vi "goto2.vi"() -> ()   [LabVIEW 2016]
uses:
  <vilib>/addons/control/pid/pid.llb/PID (DBL).vi
  <vilib>/addons/control/pid/NI_PID_pid.lvlib
panel:
  in  "max pwm\ndist condition":dbl=500.0 format="%#_13g"
  in  "max  pwm\nmultiplier":dbl=1.0 format="%#_13g"
  in  "stop dist\ncondition":dbl=100.0 format="%#_13g"
  in  "PID gains":T1={"proportional gain (Kc)"=1.0, "integral time (Ti, min)"=0.01, "derivative time (Td, min)"=0.0} {"derivative time (Td, min)" format="%.3f"; "integral time (Ti, min)" format="%.3f"; "proportional gain (Kc)" format="%.3f"}
  in  "gain":dbl=0.01 format="%#_13g"
  out "speed out":dbl[](array[numeric])
  in  "Pose":dbl[](array[numeric])
  in  "Target":dbl[](array[numeric])
  # "X"
  # "Y"
  # "W"
  # "X"
  # "vx"
  # "Y"
  # "vy"
  # "W"
  # "vw"
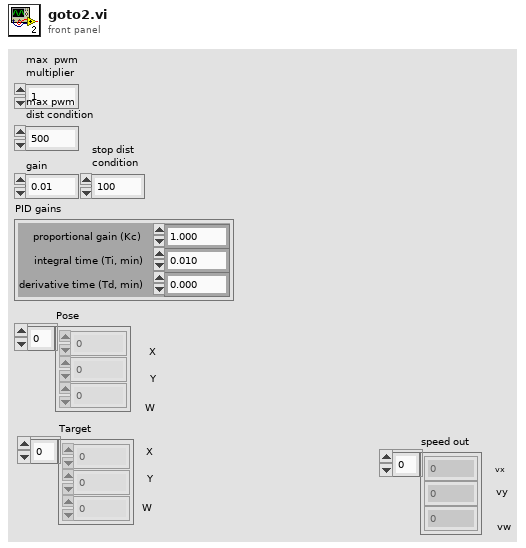
[diagram p1: front panel]
types:
  T1 = cluster{"proportional gain (Kc)":dbl, "integral time (Ti, min)":dbl, "derivative time (Td, min)":dbl}
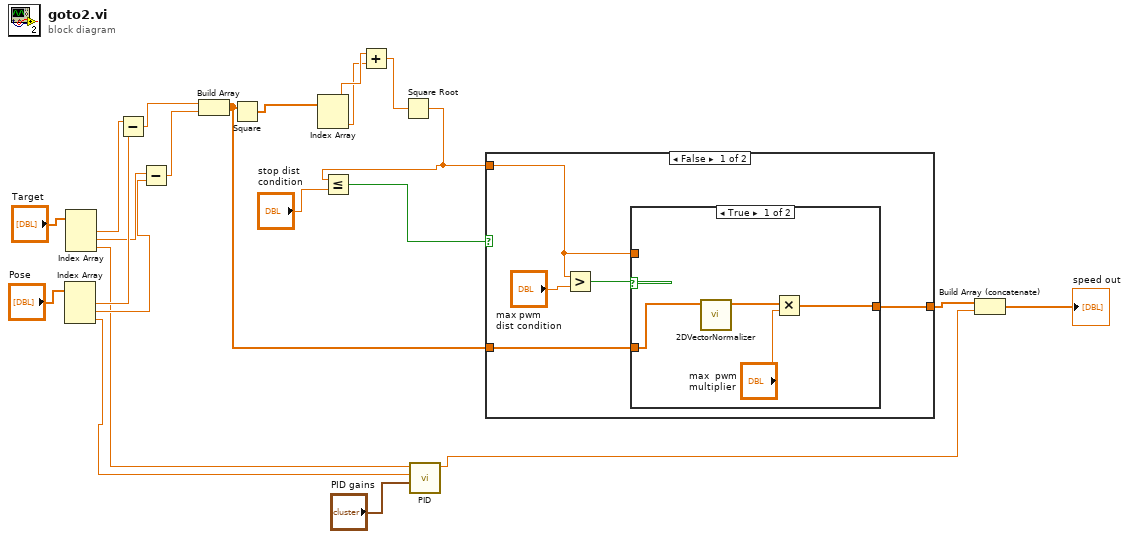
[diagram p0: block diagram]
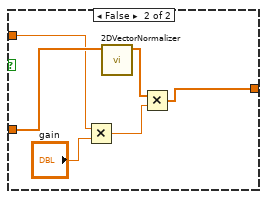
[diagram p2: hidden frame]
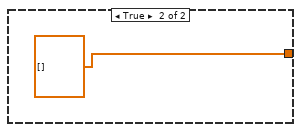
[diagram p3: hidden frame]
diagram:
  n1 = Index Array(array="Pose") -> (element #1=w19:dbl, element #2=w17:dbl, element #3=w5:dbl)  [unwired: 3 in]
  n2 = Index Array(array="Target") -> (element #1=w20:dbl, element #2=w18:dbl, element #3=w6:dbl)  [unwired: 3 in]
  n3 = Subtract(x=w20, y=w19) -> (x-y=w13:dbl)
  n4 = Subtract(x=w18, y=w17) -> (x-y=w14:dbl)
  n5 = Build Array(w13, w14) -> (w10:dbl[])
  n6 = Square(x=w10) -> (x^2=w9:dbl[])
  n7 = Index Array(array=w9) -> (element #1=w12:dbl, element #2=w11:dbl)  [unwired: 2 in]
  n8 = Add(x=w12, y=w11) -> (x+y=w8:dbl)
  n9 = Square Root(x=w8) -> (sqrt(x)=w7:dbl)
  n10 = Less Or Equal?(x=w7, y="stop dist\ncondition") -> (x <= y?=w15:bool)
  n11 = call-poly <vilib>:"PID.vi"("PID gains"="PID gains", "process variable"=w5, "setpoint"=w6) -> ("output"=w2:dbl)  [unwired: 7 in, 1 out]
  n12 = case shown="False" w15 {
    tunnel: w7 -> [w24 _]
    tunnel: [w23 dbl[] [] ("appended array")] -> w3
    tunnel: w10 -> [w25 _]
    frame False {
      n13 = Greater?(x=w24, y="max pwm\ndist condition") -> (0:w26:bool)
      n14 = case shown="True" w26 {
        tunnel: w25 -> [w31 w37]
        tunnel: w24 -> [_ w36]
        tunnel: [w29 w32] -> w23
        frame True {
          n15 = call "2DVectorNormalizer.vi"("2D vector"=w31) -> ("2D vector 2"=w30:dbl[])  [unwired: 10 in]
          n16 = Multiply(x=w30, y="max  pwm\nmultiplier") -> (x*y=w29:dbl[])
        }
        frame False {
          n17 = Multiply(x=w36, y="gain") -> (x*y=w33:dbl)
          n18 = call "2DVectorNormalizer.vi"("2D vector"=w37) -> ("2D vector 2"=w34:dbl[])  [unwired: 10 in]
          n19 = Multiply(x=w34, y=w33) -> (x*y=w32:dbl[])
        }
      }
    }
    frame True {
    }
  }
  n20 = Build Array (concatenate)(w3, w2) -> (→"speed out":dbl[])
